vi "1D Cross Correlation (DBL).vi"(8 "normalization":enum32{"none", "unbiased", "biased"}(ring), 9 "algorithm":enum32{"direct", "frequency domain"}(ring)=enum."frequency domain", 10 "Y":dbl[](array[numeric]), 11 "X":dbl[](array[numeric])) -> (0 "error":i32, 3 "Rxy":dbl[](array[numeric]))   [LabVIEW 2020, in "NI_AALPro.lvlib"]
doc: "Computes the cross correlation of the input sequences <B>X</B> and <B>Y</B>. Wire data to the <B>X</B> and <B>Y</B> inputs to determine the polymorphic instance to use or manually select the instance."
uses:
  <vilib>/Analysis/NI_AALPro.lvlib
  <resource>/lvanlys.dll
panel:
  # "1D CrossCorrelation (DBL)"
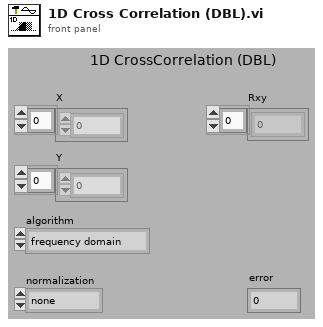
[diagram p1: front panel]
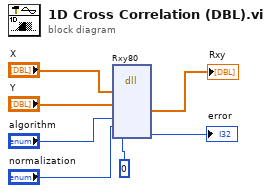
[diagram p0: block diagram]
diagram:
  n1 = dll-call lib="e:/builds/penguin/labview/branches/2020/dev/dist/resource/lvanlys.*" fn="Rxy80"("X"="X", "Y"="Y", "algorithm"="algorithm", "norm"="normalization", "error"=0) -> ("Rxy"=→"Rxy":dbl[], "error"=→"error":i32)  [unwired: 9 in, 2 out]
